vi "get_memory_usage.vi"(8 "error in (no error)":errorcluster, 11 "Lua in":refnum<class "Lua.lvclass">) -> (0 "error out":errorcluster, 2 "bytes":i64, 3 "Lua out":refnum<class "Lua.lvclass">)   [LabVIEW 2020, in "Lua for LabVIEW.lvlib" / "Lua.lvclass"]
uses:
  Lua.lvclass
  Lua.lvclass/Lua.ctl
  lib/lua.dll/types/LUA_GC.ctl
  lib/lua.dll/lua.dll.lvlib
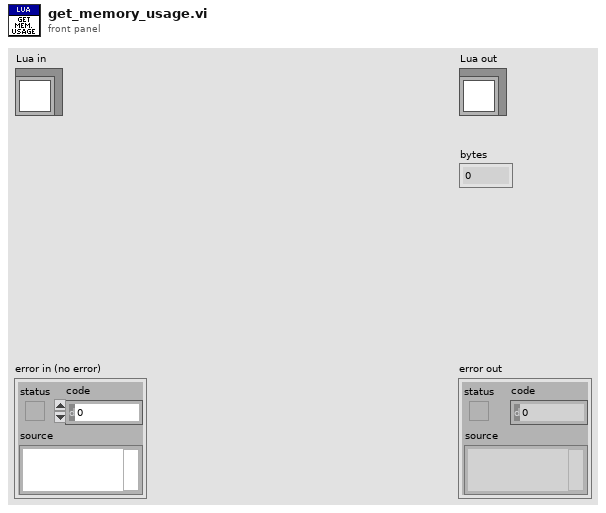
[diagram p1: front panel]
types:
  T1 = typedef "lua.dll.lvlib/LUA_GC.ctl" = enum32{"LUA_GCSTOP", "LUA_GCRESTART", "LUA_GCCOLLECT", "LUA_GCCOUNT", "LUA_GCCOUNTB", "LUA_GCSTEP", "LUA_GCSETPAUSE", "LUA_GCSETSTEPMUL", "LUA_GCSETMAJORINC", "LUA_GCISRUNNING", "LUA_GCGEN", "LUA_GCINC"}
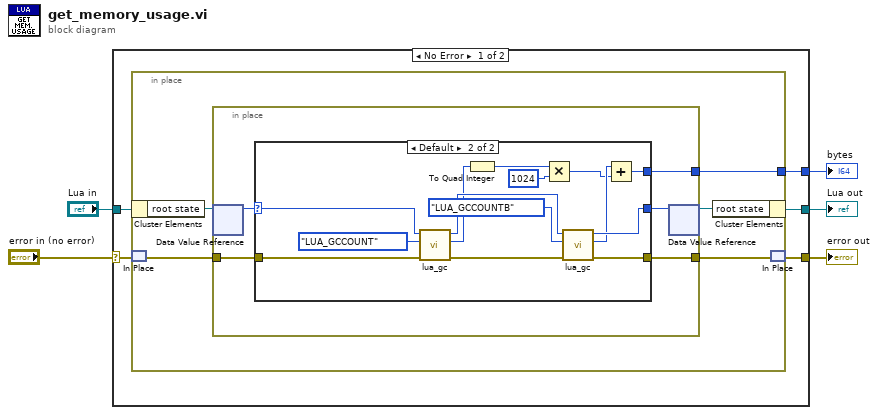
[diagram p0: block diagram]
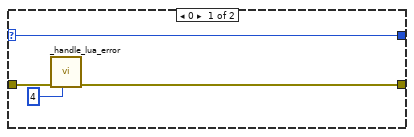
[diagram p2: hidden frame]
diagram:
  n1 = case shown="No Error" "error in (no error)" {
    selector: "error in (no error)" -> [w9 w40]
    tunnel: [w8 w40] -> w2
    tunnel: [w7 w39] -> w3
    tunnel: "Lua in" -> [w10 w39]
    tunnel: [w6 _] -> w1
    frame No Error {
      n2 = in-place {
        in-place-border: [w11] -> w6
        n3 = in-place-cluster #1(w10) -> ("root state"=w13:refnum<data-value>)
        n4 = in-place-match #2(w9) -> (w15:errorcluster)
        n5 = in-place {
          in-place-border: w15 -> [w20]
          in-place-border: [w19] -> w14
          in-place-border: [w16] -> w11
          n6 = in-place-dvr #3(w13) -> (w18:u64)  [unwired: 1 out]
          n7 = case shown="Default" w18 {
            selector: w18 -> [w24 w38]
            tunnel: [w24 w33] -> w17
            tunnel: w20 -> [w21 w37]
            tunnel: [w22 w34] -> w19
            tunnel: [_ w25] -> w16
            frame 0 {
              n8 = call "_handle_lua_error.vi"("lua status"=4 ("lua_load errcode"), "error in (no error)"=w21) -> ("error out"=w22:errorcluster)  [unwired: 9 in]
            }
            frame Default {
              n9 = call "lua_gc.vi"("error in (no error)"=w37, "what"=LUA_GC."LUA_GCCOUNT", "lua_state_p"=w38) -> ("error out"=w35:errorcluster, "result"=w30:i32, "lua_state_p out"=w36:u64)  [unwired: 6 in]
              n10 = To Quad Integer(1:w30) -> (0:w28:i64)
              n11 = Multiply(x=w28, y=i64 1024) -> (x*y=w26:i64)
              n12 = call "lua_gc.vi"("error in (no error)"=w35, "what"=LUA_GC."LUA_GCCOUNTB", "lua_state_p"=w36) -> ("error out"=w34:errorcluster, "result"=w27:i32, "lua_state_p out"=w33:u64)  [unwired: 6 in]
              n13 = Add(x=w27, y=w26) -> (x+y=w25:i64)
            }
          }
          n14 = in-place-dvr #3(w17) -> (w12:refnum<data-value>)  [unwired: 1 out]
        }
        n15 = in-place-cluster #1("root state"=w12) -> (w7:refnum<class "Lua.lvclass">)
        n16 = in-place-match #2(w14) -> (w8:errorcluster)
      }
    }
    frame Error {
    }
  }
  "error out" <- w2
  "Lua out" <- w3
  "bytes" <- w1
